vi "parseNfilterSVNLog.vi"(9 "changelogIn":string, 10 "svnLog":string, 11 "associatedVIs":string[](array[string])) -> (1 "relevantChangelogOut":string)   [LabVIEW 2021]
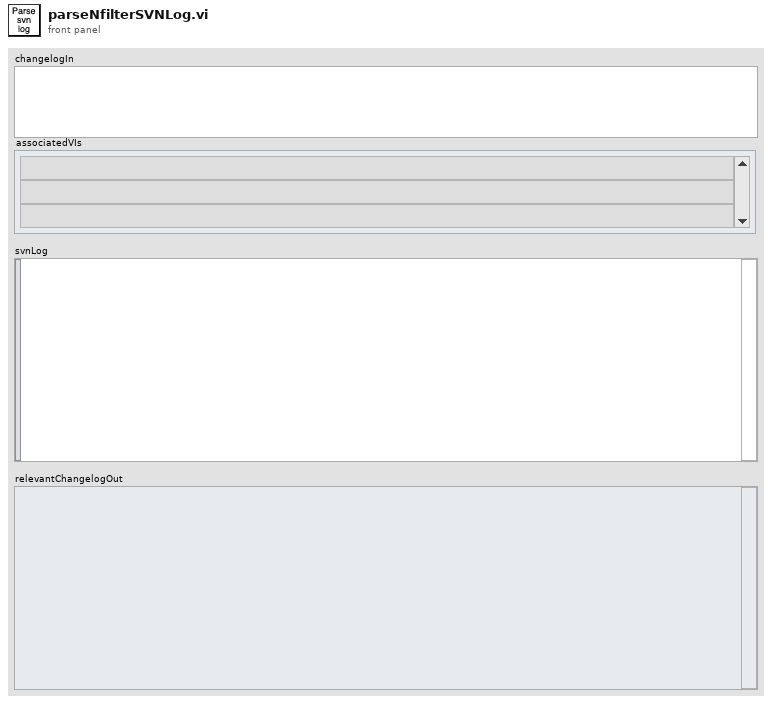
[diagram p1: front panel]
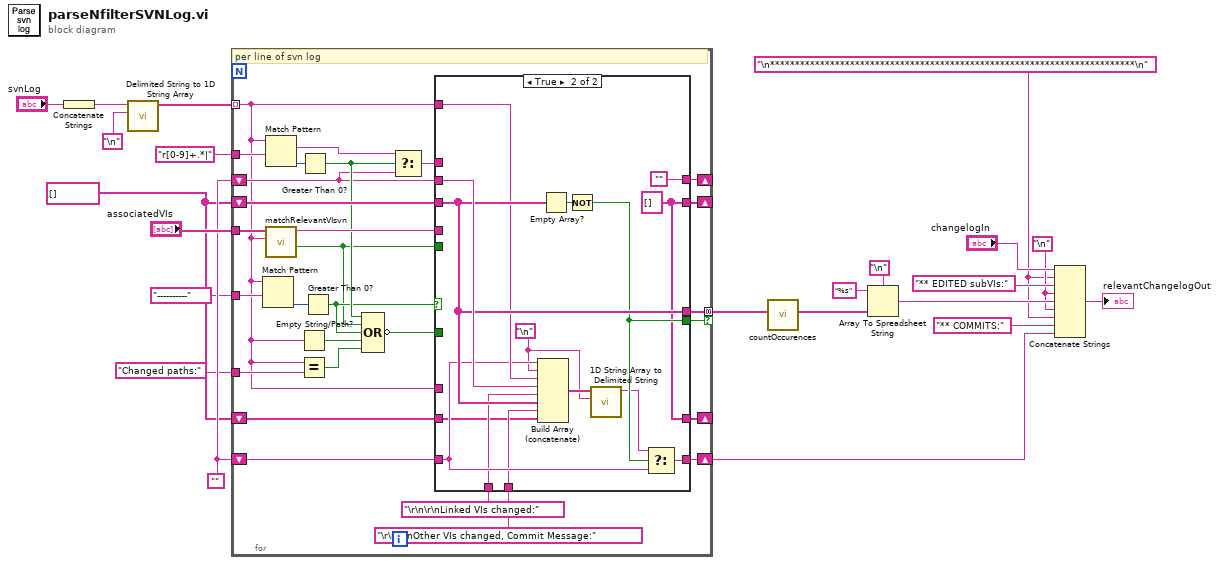
[diagram p0: block diagram]
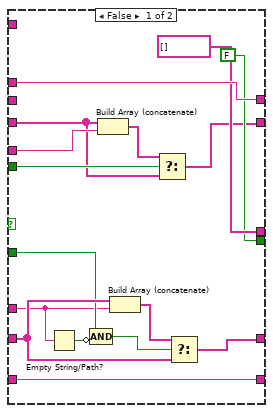
[diagram p2: hidden frame]
diagram:
  w1 = "\n*************************************************************************\n" ("string")
  w4 = string[] []
  w11 = ""
  w6 = "\n" ("delimiter (Tab)")
  n1 = Concatenate Strings("svnLog") -> (w20:string)
  n2 = call <vilib>:"Delimited String to 1D String Array.vi"("delimiter"="\n", "delimited string"=w20) -> ("string array"=w13:string[])  [unwired: 9 in]
  n3 = for {
    tunnel: w13 -> [w25] mode=indexing
    shift-right: [w47] -> _
    shift-left: w11 -> [w34]
    tunnel: "associatedVIs" -> [w45]
    shift-right: [w36] -> _
    shift-left: w4 -> [w23]
    shift-right: [w42] -> _
    shift-left: w4 -> [w44]
    shift-right: [w32] -> w10
    shift-left: w11 -> [w33]
    tunnel: "r[0-9]+.*|" ("regular expression") -> [w48]
    tunnel: "----------" ("regular expression") -> [w40]
    tunnel: [w35] -> w3 mode=concatenating if=w31
    tunnel: "Changed paths:" ("regular expression") -> [w29]
    # "per line of svn log"
    n4 = Match Pattern(string=w25, regular expression=w40) -> (offset past match=w39:i32)  [unwired: 1 in, 3 out]
    n5 = Match Pattern(string=w25, regular expression=w48) -> (match substring=w49:string, offset past match=w50:i32)  [unwired: 1 in, 2 out]
    n6 = call "matchRelevantVIsvn.vi"("logEntry"=w25, "associatedVIs"=w45) -> ("found"=w30:bool, "relevantPath"=w43:string)  [unwired: 8 in]
    n7 = Empty String/Path?(string/path=w25) -> (empty?=w37:bool)
    n8 = Equal?(x=w25, y=w29) -> (x = y?=w28:bool)
    n9 = Greater Than 0?(x=w50) -> (x > 0?=w41:bool)
    n10 = Greater Than 0?(x=w39) -> (x > 0?=w38:bool)
    n11 = Compound Arithmetic op=OR(w41, w30, w38, w37, w28) -> (invert w24:bool)
    n12 = Select(t=w49, s=w41, f=w34) -> (s? t:f=w46:string)
    n13 = case shown="True" w38 {
      tunnel: [w66 ""] -> w47
      tunnel: w46 -> [w66 _]
      tunnel: w44 -> [w58 w80]
      tunnel: w43 -> [w65 _]
      tunnel: [w59 w67] -> w42
      tunnel: [w56 w67] -> w36
      tunnel: [string[] [] w80] -> w35
      tunnel: w34 -> [_ w81]
      tunnel: w25 -> [_ w73]
      tunnel: w33 -> [w63 w72]
      tunnel: [w63 w76] -> w32
      tunnel: [FALSE w75] -> w31
      tunnel: w30 -> [w61 _]
      tunnel: "\r\n\r\nOther VIs changed, Commit Message:" ("element") -> [_ w70]
      tunnel: "\r\n\r\nLinked VIs changed:" ("element") -> [_ w69]
      tunnel: w25 -> [w51 _]
      tunnel: w24 -> [w54 _]
      tunnel: w23 -> [w55 w68]
      frame False {
        n14 = Empty String/Path?(string/path=w51) -> (empty?=w52:bool)
        n15 = Compound Arithmetic op=AND(w54, invert w52) -> (w53:bool)
        n16 = Build Array (concatenate)(w58, w65) -> (w60:string[])
        n17 = Build Array (concatenate)(w55, w51) -> (w57:string[])
        n18 = Select(t=w60, s=w61, f=w58) -> (s? t:f=w59:string[])
        n19 = Select(t=w57, s=w53, f=w55) -> (s? t:f=w56:string[])
      }
      frame True {
        w71 = "\n"
        w67 = string[] []
        n20 = Build Array (concatenate)(w72, w71, w73, w81, w69, w80, w70, w68) -> (w78:string[])
        n21 = Empty Array?(array=w80) -> (empty?=w79:bool)
        n22 = Not(x=w79) -> (.not. x?=w75:bool)
        n23 = call <vilib>:"1D String Array to Delimited String.vi"("delimiter"=w71, "string array"=w78) -> ("delimited string"=w74:string)  [unwired: 9 in]
        n24 = Select(t=w74, s=w75, f=w72) -> (s? t:f=w76:string)
      }
    }
  }
  n25 = call "countOccurences.vi"("modifiedPaths"=w3) -> ("frequencyXmodifiedPaths"=w2:string[])  [unwired: 10 in]
  n26 = Array To Spreadsheet String(delimiter (Tab)="\n", array=w2, 3:"%s" ("format string")) -> (spreadsheet string=w15:string)
  n27 = Concatenate Strings("changelogIn", w1, "** EDITED subVIs:" ("string"), w6, w15, w6, w1, "** COMMITS:" ("string"), w10) -> (→"relevantChangelogOut":string)
